vi "Process.vi"(8 "error in":errorcluster, 11 "Plugin in":refnum<class "Sequencer with Output Values.lvclass">) -> (0 "error out":errorcluster, 3 "Plugin out":refnum<class "Sequencer with Output Values.lvclass">)   [LabVIEW 2024, in "Sequencer with Output Values.lvlib" / "Sequencer with Output Values.lvclass"]
uses:
  Sequencer with Output Values.lvclass
  C:/Program Files/National Instruments/LabVIEW 2024/vi.lib/FlexLogger/SDK/PluginSDK.lvlibp/PEFClasses/SDK/Plugin/Plugin.lvclass
  Sequencer with Output Values.lvclass/Sequencer with Output Values.ctl
  <vilib>/FlexLogger/SDK/PluginSDK.lvlibp/PEFClasses/SDK/Plugin/DataHelpers/Write 1D DBL (NChan 1Sample).vi
  <vilib>/FlexLogger/SDK/PluginSDK.lvlibp/PEFClasses/SDK/Plugin/DataHelpers/Write 1D Bool (NChan 1 Sample).vi
  Global Strings.vi
  <vilib>/FlexLogger/SDK/PluginSDK.lvlibp/PEFClasses/SDK/Plugin/ParameterAccess/Write String.vi
  <vilib>/FlexLogger/SDK/PluginSDK.lvlibp/PEFClasses/SDK/Plugin/Plugin.lvclass
  <vilib>/FlexLogger/SDK/PluginSDK.lvlibp
  C:/Program Files/National Instruments/LabVIEW 2024/vi.lib/FlexLogger/SDK/PluginSDK.lvlibp/PEFClasses/SDK/Processing Element/Processing Element.lvclass
  C:/dev/niflexlogger-plugins/plugins/Sequencer with Output Values/source/Sequencer with Output Values/Sequencer with Output Values.lvclass
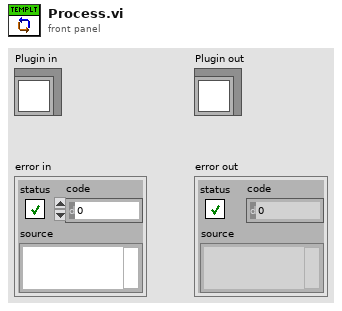
[diagram p1: front panel]
types:
  T1 = typedef "Sequencer with Output Values.lvlib/Sequencer with Output Values.lvclass/Params.ctl" = cluster{"Step Values":T2[], "Only Execute When Test Running":bool, "Reset Sequence When Test Starts":bool, "Current Sequence ID":u32, "Total Iterations":u32, "Last Timestamp":dbl, "Number of Sequence Steps":i32, "Num of Analog Channels":i32, "Num of Digital Channels":i32, "Delay Before Starting Sequence":dbl, "Changed":bool}
  T2 = typedef "Sequencer with Output Values.lvlib/Sequencer with Output Values.lvclass/Step Settings.ctl" = cluster{"Duration":dbl, "Mode":string, "Delay Between Values":dbl, "Analog Values":string[], "Digital Values":string[]}
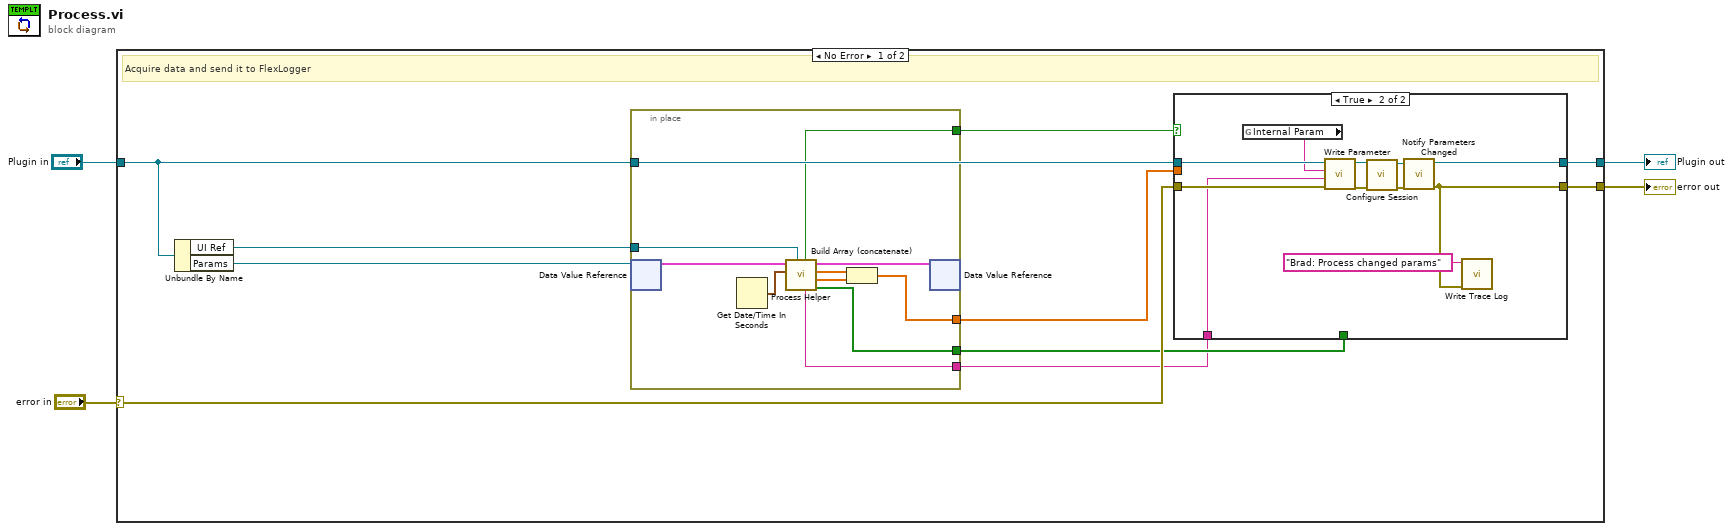
[diagram p0: block diagram]
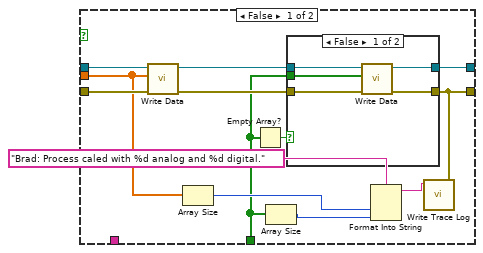
[diagram p2: hidden frame]
diagram:
  n1 = case shown="No Error" "error in" {
    selector: "error in" -> [w14 w56]
    tunnel: [w10 w57] -> w4
    tunnel: "Plugin in" -> [w8 w57]
    tunnel: [w9 w56] -> w1
    frame No Error {
      # "Acquire data and send it to FlexLogger"
      n2 = Unbundle By Name(w8) -> ("UI Ref"=w5:refnum<vi>, "Params"=w13:refnum<data-value>)
      n3 = in-place {
        in-place-border: [w48] -> w12
        in-place-border: [w51] -> w11
        in-place-border: w8 -> [_]
        in-place-border: [w53] -> w7
        in-place-border: [w47] -> w6
        in-place-border: w5 -> [w46]
        n4 = in-place-dvr #1(w13) -> (w55:T1)  [unwired: 1 out]
        n5 = Get Date/Time In Seconds() -> (seconds since 1Jan1904=w54:timestamp)
        n6 = call "Process Helper.vi"("UI Ref"=w46, "current time"=w54, "Settings in"=w55) -> ("Digital Values to Write"=w51:bool[], "Analog Values to Write"=w49:dbl[], "Sequence State Channels to Write"=w50:dbl[], "Settings out"=w52:T1, "New Settings"=w47:string, "Changed"=w53:bool)  [unwired: 3 in]
        n7 = Build Array (concatenate)(w50, w49) -> (w48:dbl[])
        n8 = in-place-dvr #1(w52) -> ()  [unwired: 2 out]
      }
      n9 = case shown="True" w7 {
        tunnel: w14 -> [w27 w44]
        tunnel: w12 -> [w18 _]
        tunnel: w11 -> [w16 _]
        tunnel: [w26 w36] -> w10
        tunnel: [w19 w42] -> w9
        tunnel: w8 -> [w22 w45]
        tunnel: w6 -> [_ w35]
        frame False {
          n10 = call-poly <vilib>:"Write Data.vi"("error in (no error)"=w27, "Data"=w18, "Plugin in"=w22) -> ("error out"=w24:errorcluster, "Plugin out"=w25:refnum<class "Sequencer with Output Values.lvclass">)  [unwired: 7 in]
          n11 = Array Size(array=w18) -> (size(s)=w17:i32)
          n12 = Empty Array?(array=w16) -> (empty?=w23:bool)
          n13 = Array Size(array=w16) -> (size(s)=w15:i32)
          n14 = case shown="False" w23 {
            tunnel: w25 -> [w32 w34]
            tunnel: w24 -> [w31 w33]
            tunnel: [w30 w34] -> w26
            tunnel: [w29 w33] -> w19
            tunnel: w16 -> [w28 _]
            frame False {
              n15 = call-poly <vilib>:"Write Data.vi"("error in (no error)"=w31, "Data"=w28, "Plugin in"=w32) -> ("error out"=w29:errorcluster, "Plugin out"=w30:refnum<class "Sequencer with Output Values.lvclass">)  [unwired: 7 in]
            }
            frame True {
            }
          }
          n16 = Format Into String(format string="Brad: Process caled with %d analog and %d digital.", w17, w15) -> (resulting string=w20:string)  [unwired: 2 in, 1 out]
          n17 = call <vilib>:"Write Trace Log.vi"("error in (no error)"=w19, "Message"=w20) -> ()  [unwired: 9 in, 1 out]
        }
        frame True {
          n18 = global read "Global Strings.vi" "Internal Param"() -> (w43:string)
          n19 = call-poly <vilib>:"Write Parameter.vi"("error in (no error)"=w44, "Value"=w35, "Name"=w43, "Plugin in"=w45) -> ("error out"=w40:errorcluster, "Plugin out"=w39:refnum<class "Sequencer with Output Values.lvclass">)  [unwired: 6 in]
          n20 = call-dynamic "Configure Session.vi"("error in"=w40, "Plugin in"=w39) -> ("error out"=w37:errorcluster, "Plugin out"=w38:refnum<class "Sequencer with Output Values.lvclass">)  [unwired: 8 in]
          n21 = call <vilib>:"Notify Parameters Changed.vi"("error in (no error)"=w37, "Plugin in"=w38) -> ("error out"=w42:errorcluster, "Plugin out"=w36:refnum<class "Sequencer with Output Values.lvclass">)  [unwired: 8 in]
          n22 = call <vilib>:"Write Trace Log.vi"("error in (no error)"=w42, "Message"="Brad: Process changed params") -> ()  [unwired: 9 in, 1 out]
        }
      }
    }
    frame Error {
    }
  }
  "error out" <- w1
  "Plugin out" <- w4
